vi "ShifterHax.vi"(10 "Automatic Shifting":bool, 11 "Manual Shift Low":bool) -> ()   [LabVIEW 2012]
uses:
  <vilib>/Rock Robotics/WPI/Solenoid/Deprecated/WPI_SolenoidSetBool.vi
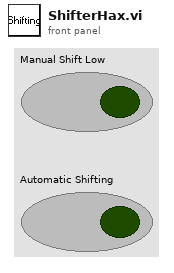
[diagram p1: front panel]
types:
  T1 = typedef "WPI_SolenoidDevRef.ctl" = cluster{"DevStatus":errorcluster, "Solenoid Module":T2, "Forward Solenoid Channel":T3, "Reverse Solenoid Channel":T3}
  T2 = typedef "FPGA_TypedefSolenoidModule.ctl" = enum16{"Solenoid Module 1", "Solenoid Module 2"}
  T3 = typedef "WPI_SolenoidChannel.ctl" = enum8{"Solenoid 1", "Solenoid 2", "Solenoid 3", "Solenoid 4", "Solenoid 5", "Solenoid 6", "Solenoid 7", "Solenoid 8", "Invalid"}
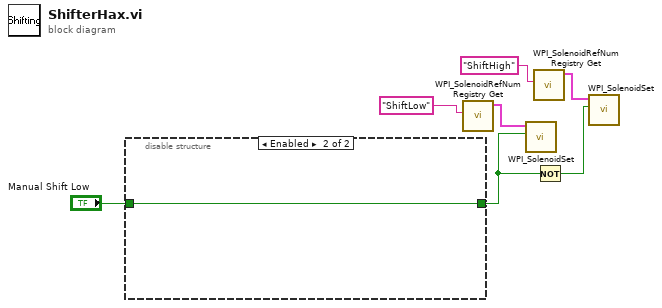
[diagram p0: block diagram]
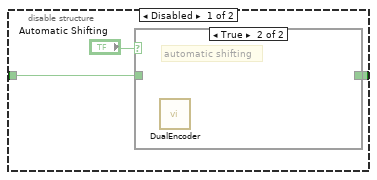
[diagram p2: hidden frame]
diagram:
  n1 = disable-structure shown="Enabled" {
    disable-tunnel: [w9 w12] -> w2
    disable-tunnel: "Manual Shift Low" -> [w8 w12]
    frame Disabled {
      n2 = case shown="True" "Automatic Shifting" {
        tunnel: [w11 _] -> w9
        tunnel: w8 -> [w11 _]
        frame False {
          # "normal manual shifting"
        }
        frame True {
          # "automatic shifting"
          n3 = call "DualEncoder.vi"() -> ()  [unwired: 7 in, 5 out]
        }
      }
    }
    frame Enabled {
    }
  }
  n4 = call <vilib>:"WPI_SolenoidRefNum Registry Get.vi"("refnum name"="ShiftLow") -> ("SolenoidDevRef"=w7:T1)  [unwired: 9 in, 1 out]
  n5 = call-poly <vilib>:"WPI_SolenoidSet.vi"("Value"=w2, "SolenoidDevRef"=w7) -> ()  [unwired: 1 in, 9 out]
  n6 = call <vilib>:"WPI_SolenoidRefNum Registry Get.vi"("refnum name"="ShiftHigh") -> ("SolenoidDevRef"=w6:T1)  [unwired: 9 in, 1 out]
  n7 = Not(x=w2) -> (.not. x?=w5:bool)
  n8 = call-poly <vilib>:"WPI_SolenoidSet.vi"("Value"=w5, "SolenoidDevRef"=w6) -> ()  [unwired: 1 in, 9 out]
